vi "UI_Lubricate_Unit_Test.vi"() -> ()   [LabVIEW 2014]
panel:
  in  "修改":bool
  in  "试验轴承单元回油过滤器堵塞":bool caption="回油过滤器堵塞"
  in  "试验轴承单元循环回路过滤器堵塞":bool caption="循环回路过滤器堵塞"
  in  "试验轴承单元供油过滤器堵塞":bool caption="供油过滤器堵塞"
  in  "试验轴承单元油箱2液位过低":bool caption="油箱2液位过低"
  in  "试验轴承单元油箱2液位过高":bool caption="油箱2液位过高"
  in  "试验轴承单元油箱1液位过低":bool caption="油箱1液位过低"
  in  "试验轴承单元油箱1液位过高":bool caption="油箱1液位过高"
  in  "试验轴承单元加热装置异常":bool caption="加热装置异常"
  out "传感器出油温度":dbl(graph)
  in  "退出":bool
  out "油箱1油温":dbl(graph)
  out "润滑油温度":dbl(graph)
  out "供油压力":dbl(graph)
  out "供油流量":dbl(graph)
  out "油箱2油温":dbl(graph)
  out "实验轴承单元调试状态":bool
  in  "开始调试":bool
  in  "供油润滑油温度T":u16
  in  "供油流量L":u16
  # "试验轴承润滑单元独立调试"
  # "监测参数"
  # "采集卡采集数据"
  # "当前值"
  # "℃"
  # "单元系统数据"
  # "报警信息"
  # "当前值"
  # "当前值"
  # "当前值"
  # "℃"
  # "℃"
  # "KN"
  # "当前值"
  # "当前值"
  # "L"
  # "℃"
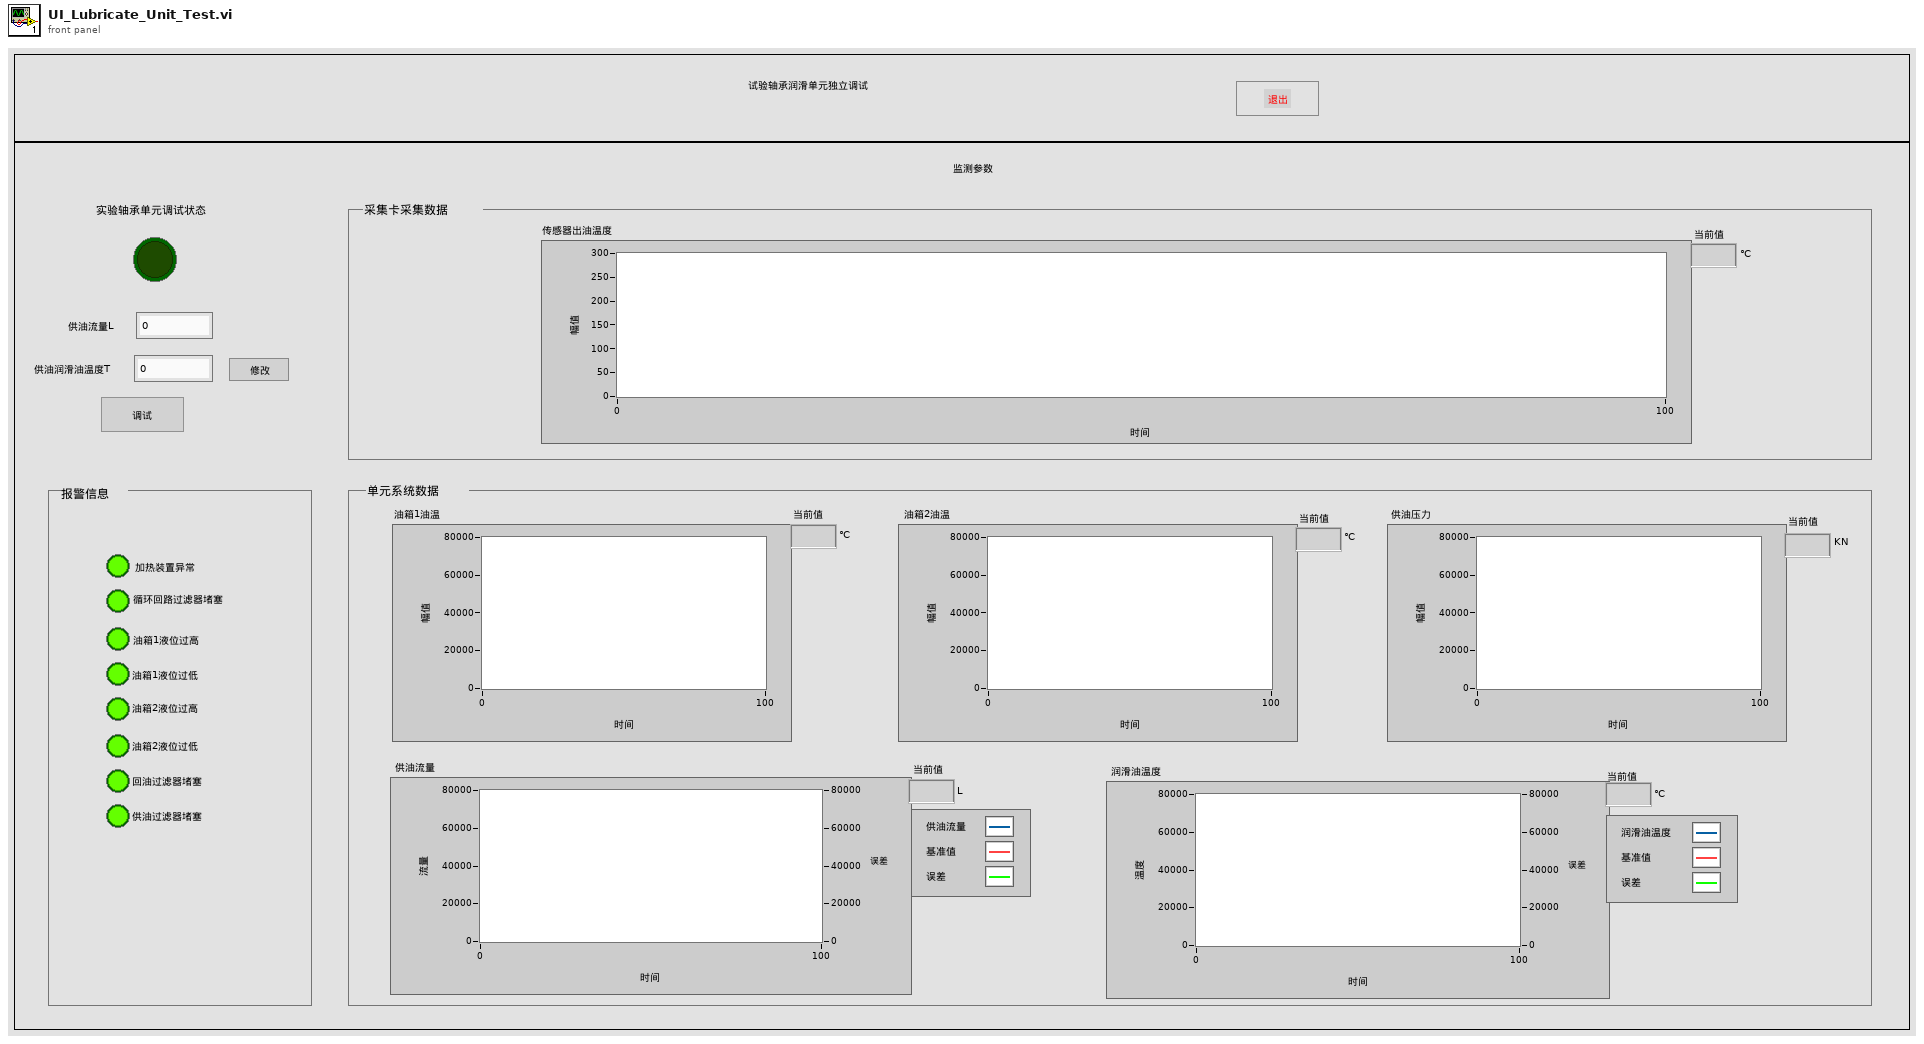
[diagram p1: front panel]
types:
  T1 = cluster{"径向油缸加载压力":u16, "轴向油缸加载压力":u16, "油箱1油液温度":u16, "润滑油温度":u16, "油箱2油液温度":u16, "试验轴承供油压力":u16, "试验轴承供油流量":u16, "陪试轴承供油流量":u16, "陪试轴承供油压力":u16, "陪试轴承供油温度":u16, "液压子系统状态字":cluster{"加载单元":cluster{"供油过滤器堵塞报警":bool, "回油过滤器堵塞报警":bool, "液位过高报警":bool, "液位过低报警":bool}, "试验轴承单元":cluster{"加热装置异常报警":bool, "油箱1液位过高报警":bool, "油箱1液位过低报警":bool, "油箱2液位过高报警":bool, "油箱2液位过低报警":bool, "供油过滤器堵塞报警":bool, "循环回路过滤器堵塞报警":bool, "回油过滤器堵塞报警":bool}, "陪试轴承单元":cluster{"供油过滤器1堵塞报警":bool, "供油过滤器2堵塞报警":bool, "回油过滤器堵塞报警":bool, "油箱液位过高报警":bool, "油箱液位过低报警":bool}}}
  T2 = cluster{"时间":timestamp, "陪试轴承润滑单元出油温度1":sgl[], "陪试轴承润滑单元出油温度2":sgl[], "轴承外圈温度":sgl[], "出油温度":sgl[], "摩擦力1":sgl[], "摩擦力2":sgl[], "径向油缸力":sgl[], "轴向油缸力":sgl[], "转速":sgl[]}
  T3 = cluster{"加热装置异常报警":bool, "油箱1液位过高报警":bool, "油箱1液位过低报警":bool, "油箱2液位过高报警":bool, "油箱2液位过低报警":bool, "供油过滤器堵塞报警":bool, "循环回路过滤器堵塞报警":bool, "回油过滤器堵塞报警":bool}
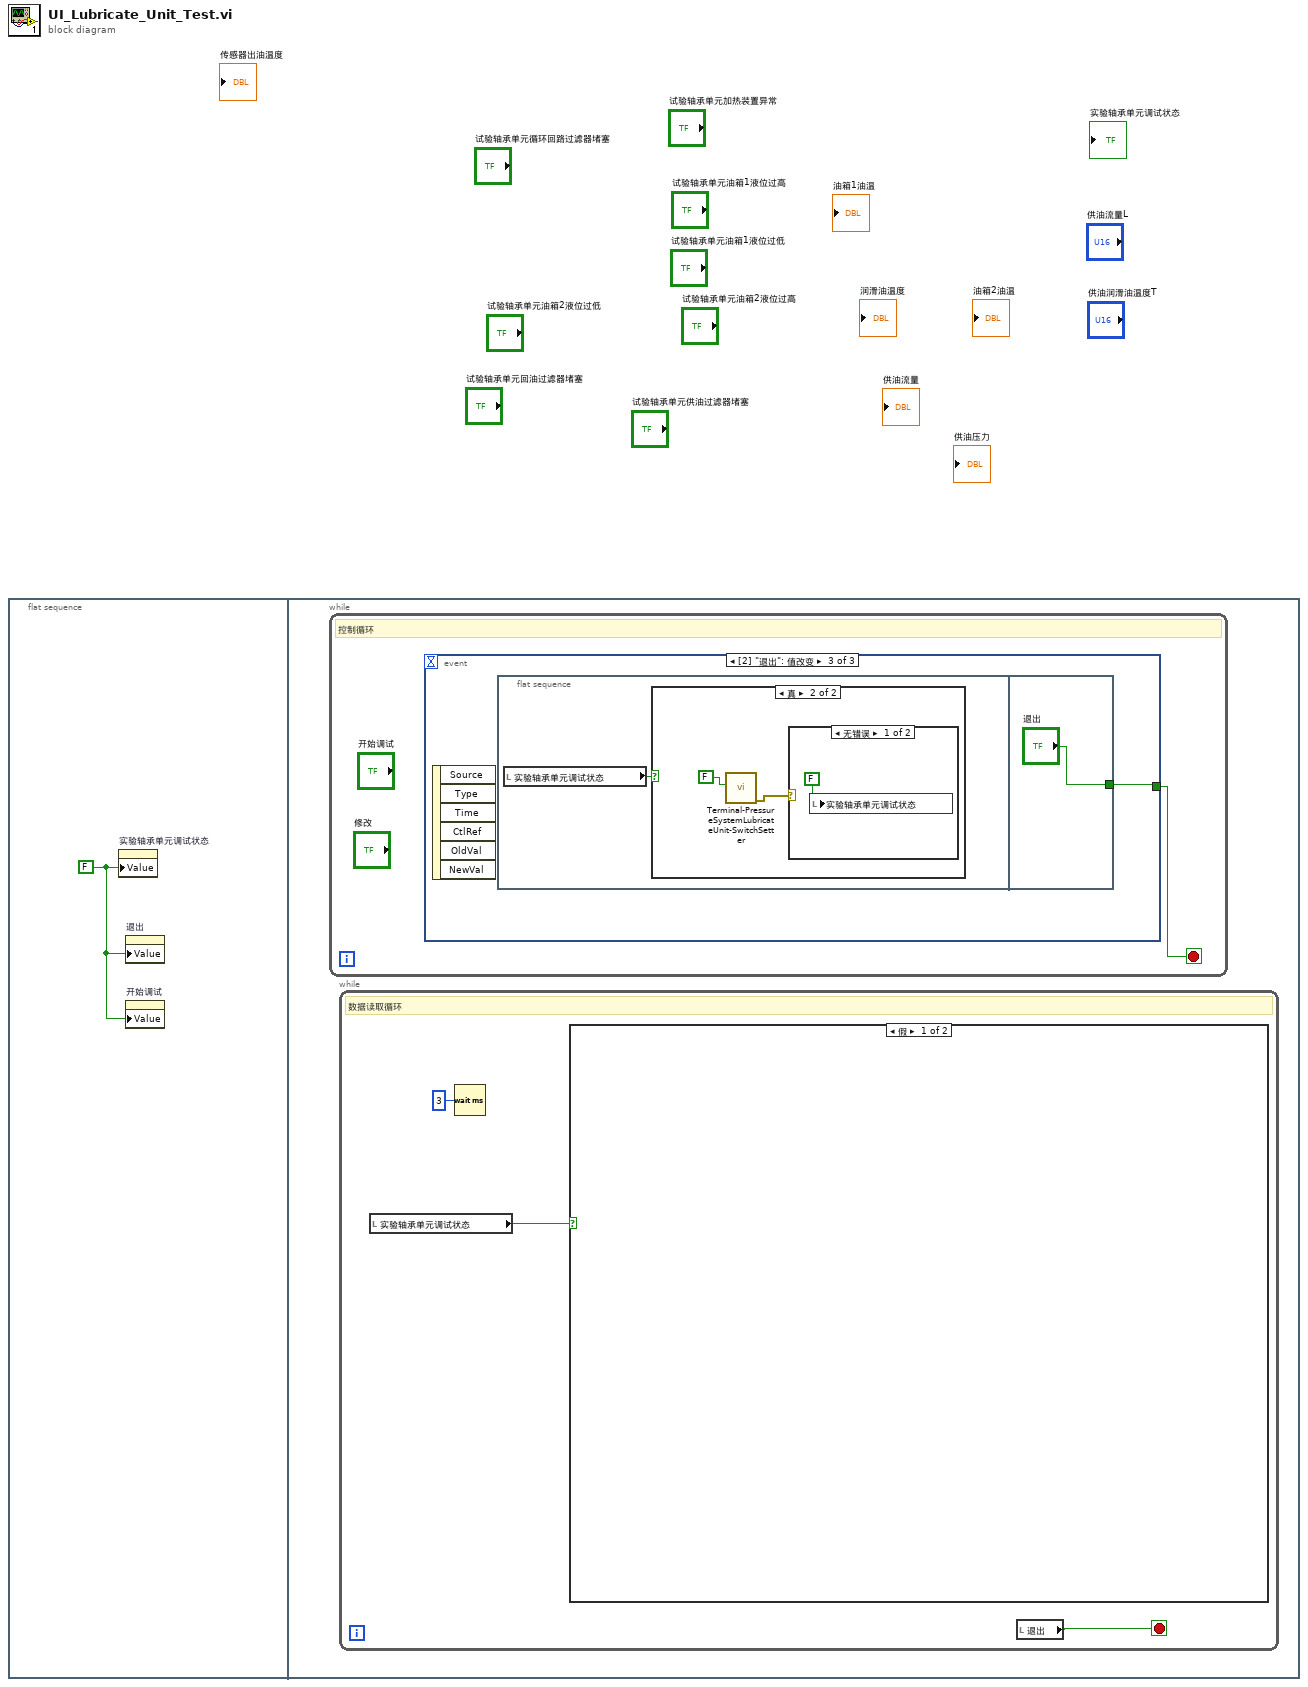
[diagram p0: block diagram]
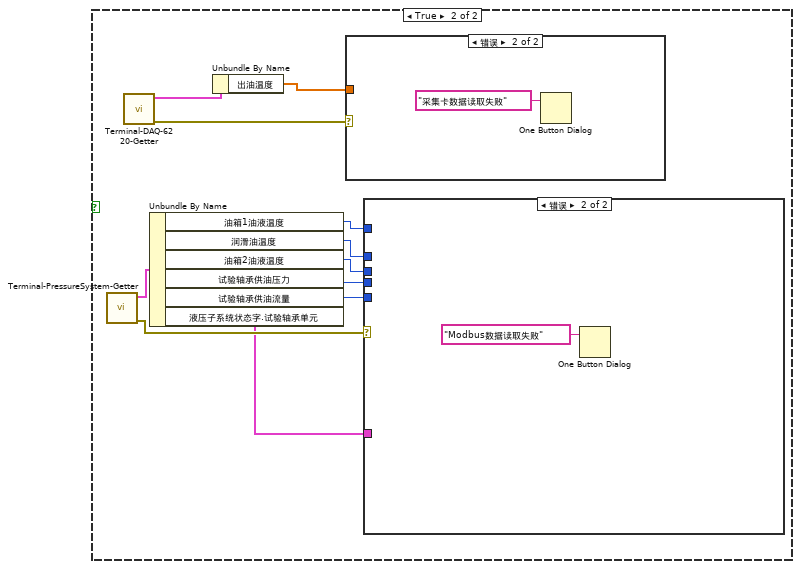
[diagram p2: hidden frame]
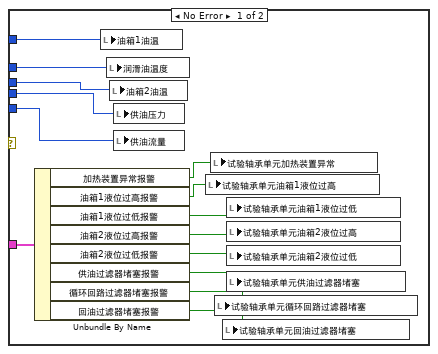
[diagram p3: hidden frame]
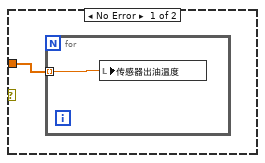
[diagram p4: hidden frame]
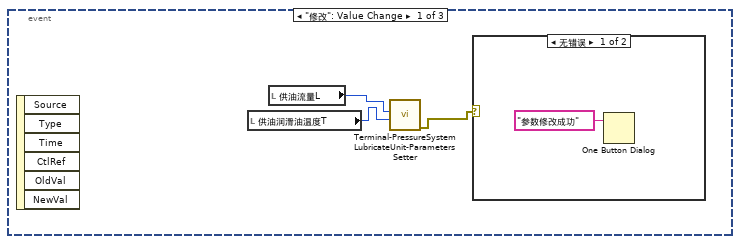
[diagram p5: hidden frame]
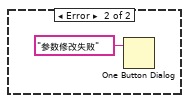
[diagram p6: hidden frame]
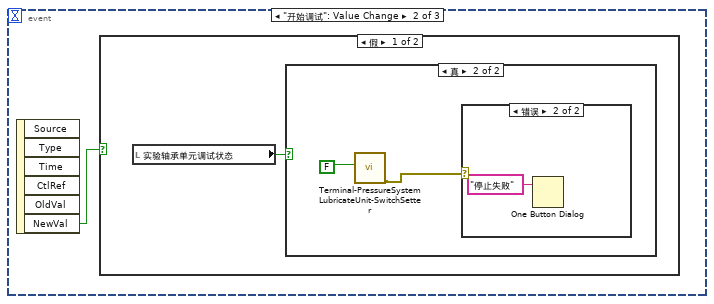
[diagram p7: hidden frame]
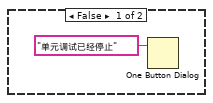
[diagram p8: hidden frame]
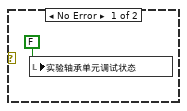
[diagram p9: hidden frame]
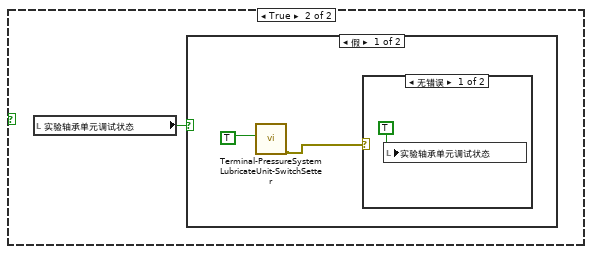
[diagram p10: hidden frame]
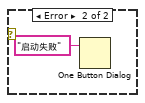
[diagram p11: hidden frame]
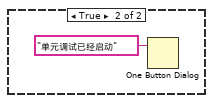
[diagram p12: hidden frame]
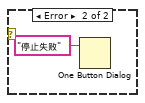
[diagram p14: hidden frame]
diagram:
  n1 = flat-sequence {
    frame #0 {
      w1 = FALSE ("实验轴承单元调试状态")
      n2 = property on="实验轴承单元调试状态" class="Bool (严格)"("Value"=w1) -> ()  [unwired: 2 in, 2 out]
      n3 = property on="退出" class="Bool (严格)"("Value"=w1) -> ()  [unwired: 2 in, 2 out]
      n4 = property on="开始调试" class="Bool (严格)"("Value"=w1) -> ()  [unwired: 2 in, 2 out]
    }
    frame #1 {
      n5 = while {
        stop <- w34 stop-if-true
        # "控制循环"
        n6 = event shown="[2] \"退出\": 值改变" {
          selector: _ -> [_ _ _]
          dyn-events: _ -> [_ _ _]
          timeout: _ -> [_ _ _]
          tunnel: [_ _ w53] -> w34
          event "修改": Value Change {
            n7 = event-data() -> ()  [unwired: 1 in, 6 out]
            n8 = local read "供油润滑油温度T"() -> (w36:u16)
            n9 = local read "供油流量L"() -> (w37:u16)
            n10 = call "Terminal-PressureSystemLubricateUnit-ParametersSetter.vi"("供油润滑温度T"=w36, "供油流量L"=w37) -> ("error out"=w35:errorcluster)  [unwired: 9 in]
            n11 = case shown="无错误" w35 {
              frame No Error {
                n12 = One Button Dialog(message="参数修改成功" ("消息")) -> ()  [unwired: 1 in, 1 out]
              }
              frame Error {
                n13 = One Button Dialog(message="参数修改失败" ("消息")) -> ()  [unwired: 1 in, 1 out]
              }
            }
          }
          event "开始调试": Value Change {
            n14 = event-data() -> ("NewVal"=w40:bool)  [unwired: 1 in, 5 out]
            n15 = case shown="假" w40 {
              frame False {
                n16 = local read "实验轴承单元调试状态"() -> (w41:bool)
                n17 = case shown="真" w41 {
                  frame False {
                    n18 = One Button Dialog(message="单元调试已经停止" ("消息")) -> ()  [unwired: 1 in, 1 out]
                  }
                  frame True {
                    n19 = call "Terminal-PressureSystemLubricateUnit-SwitchSetter.vi"("启停"=FALSE) -> ("error out"=w43:errorcluster)  [unwired: 10 in]
                    n20 = case shown="错误" w43 {
                      frame No Error {
                        n21 = local write "实验轴承单元调试状态"(FALSE) -> ()
                      }
                      frame Error {
                        n22 = One Button Dialog(message="停止失败" ("消息")) -> ()  [unwired: 1 in, 1 out]
                      }
                    }
                  }
                }
              }
              frame True {
                n23 = local read "实验轴承单元调试状态"() -> (w47:bool)
                n24 = case shown="假" w47 {
                  frame False {
                    n25 = call "Terminal-PressureSystemLubricateUnit-SwitchSetter.vi"("启停"=TRUE) -> ("error out"=w48:errorcluster)  [unwired: 10 in]
                    n26 = case shown="无错误" w48 {
                      frame No Error {
                        n27 = local write "实验轴承单元调试状态"(TRUE) -> ()
                      }
                      frame Error {
                        n28 = One Button Dialog(message="启动失败" ("消息")) -> ()  [unwired: 1 in, 1 out]
                      }
                    }
                  }
                  frame True {
                    n29 = One Button Dialog(message="单元调试已经启动" ("消息")) -> ()  [unwired: 1 in, 1 out]
                  }
                }
              }
            }
          }
          event "退出": Value Change {
            n30 = event-data() -> ()  [unwired: 1 in, 6 out]
            n31 = flat-sequence {
              tunnel: ["退出"] -> w53
              frame #0 {
                n32 = local read "实验轴承单元调试状态"() -> (w54:bool)
                n33 = case shown="真" w54 {
                  frame False {
                  }
                  frame True {
                    n34 = call "Terminal-PressureSystemLubricateUnit-SwitchSetter.vi"("启停"=FALSE) -> ("error out"=w56:errorcluster)  [unwired: 10 in]
                    n35 = case shown="无错误" w56 {
                      frame No Error {
                        n36 = local write "实验轴承单元调试状态"(FALSE) -> ()
                      }
                      frame Error {
                        n37 = One Button Dialog(message="停止失败" ("消息")) -> ()  [unwired: 1 in, 1 out]
                      }
                    }
                  }
                }
              }
              frame #1 {
              }
            }
          }
        }
      }
      n38 = while {
        stop <- w3 stop-if-true
        # "数据读取循环"
        n39 = local read "实验轴承单元调试状态"() -> (w4:bool)
        n40 = Wait (ms)(milliseconds to wait=u32 3 ("等待时间（毫秒）")) -> ()  [unwired: 1 out]
        n41 = case shown="假" w4 {
          frame False {
          }
          frame True {
            n42 = call "Terminal-PressureSystem-Getter.vi"() -> ("error out"=w12:errorcluster, "设备信息"=w11:T1)  [unwired: 9 in, 1 out]
            n43 = call "Terminal-DAQ-6220-Getter.vi"() -> ("error out"=w15:errorcluster, "6220"=w14:T2)  [unwired: 10 in]
            n44 = Unbundle By Name(w11) -> ("油箱1油液温度"=w9:u16, "润滑油温度"=w8:u16, "油箱2油液温度"=w7:u16, "试验轴承供油压力"=w6:u16, "试验轴承供油流量"=w5:u16, "液压子系统状态字.试验轴承单元"=w10:T3)
            n45 = Unbundle By Name(w14) -> ("出油温度"=w13:sgl[])
            n46 = case shown="错误" w15 {
              tunnel: w13 -> [w31 _]
              frame No Error {
                n47 = for {
                  tunnel: w31 -> [w32] mode=indexing
                  n48 = local write "传感器出油温度"(w32) -> ()
                }
              }
              frame Error {
                n49 = One Button Dialog(message="采集卡数据读取失败" ("消息")) -> ()  [unwired: 1 in, 1 out]
              }
            }
            n50 = case shown="错误" w12 {
              tunnel: w10 -> [w29 _]
              tunnel: w9 -> [w28 _]
              tunnel: w8 -> [w27 _]
              tunnel: w7 -> [w26 _]
              tunnel: w6 -> [w25 _]
              tunnel: w5 -> [w16 _]
              frame No Error {
                n51 = Unbundle By Name(w29) -> ("加热装置异常报警"=w24:bool, "油箱1液位过高报警"=w23:bool, "油箱1液位过低报警"=w22:bool, "油箱2液位过高报警"=w21:bool, "油箱2液位过低报警"=w20:bool, "供油过滤器堵塞报警"=w19:bool, "循环回路过滤器堵塞报警"=w18:bool, "回油过滤器堵塞报警"=w17:bool)
                n52 = local write "油箱1油温"(w28) -> ()
                n53 = local write "润滑油温度"(w27) -> ()
                n54 = local write "油箱2油温"(w26) -> ()
                n55 = local write "供油压力"(w25) -> ()
                n56 = local write "供油流量"(w16) -> ()
                n57 = local write "试验轴承单元油箱1液位过高"(w23) -> ()
                n58 = local write "试验轴承单元加热装置异常"(w24) -> ()
                n59 = local write "试验轴承单元循环回路过滤器堵塞"(w18) -> ()
                n60 = local write "试验轴承单元回油过滤器堵塞"(w17) -> ()
                n61 = local write "试验轴承单元油箱1液位过低"(w22) -> ()
                n62 = local write "试验轴承单元油箱2液位过高"(w21) -> ()
                n63 = local write "试验轴承单元油箱2液位过低"(w20) -> ()
                n64 = local write "试验轴承单元供油过滤器堵塞"(w19) -> ()
              }
              frame Error {
                n65 = One Button Dialog(message="Modbus数据读取失败" ("消息")) -> ()  [unwired: 1 in, 1 out]
              }
            }
          }
        }
        n66 = local read "退出"() -> (w3:bool)
      }
    }
  }
